vi "video server2.vi"() -> ()   [LabVIEW 2010]
doc: "Simple Data Server write a double precision array of a specified waveform type to the given TCP port. It does not provide any mechanism to halt the server or the client."
uses:
  <vilib>/userDefined/High Color/IMAQdx.ctl
  <vilib>/Utility/tcp.llb/UDP Multicast Open.vi
  <vilib>/vision/driver/NI_Vision_Acquisition_Software.lvlib
  <vilib>/vision/NI_Vision_Development_Module.lvlib
panel:
  in  "stop":bool
  in  "Multicast Address":string="234.5.6.7"
  in  "Send to Port":u16=58432
  in  "TTL":u16=1
  in  "Local Port":u16=58431
  in  "Compression (None)":i32(ring)=1 items=["None", "JPEG", "PACKED BINARY"]
  in  "Quality":i32=750 caption="Quality (750)"
  out "Image":T1(plugin-control)
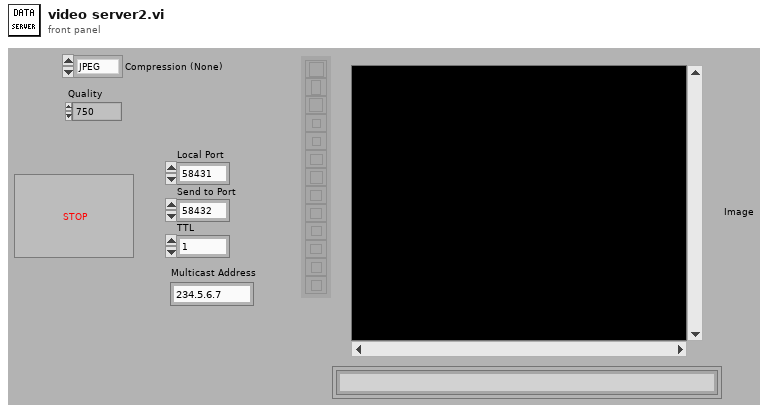
[diagram p1: front panel]
types:
  T1 = typedef "IMAQ Image.ctl" = refnum<image>
  T2 = typedef "Image Type" = u32
  T3 = typedef "IMAQdx.ctl" = refnum<k21>
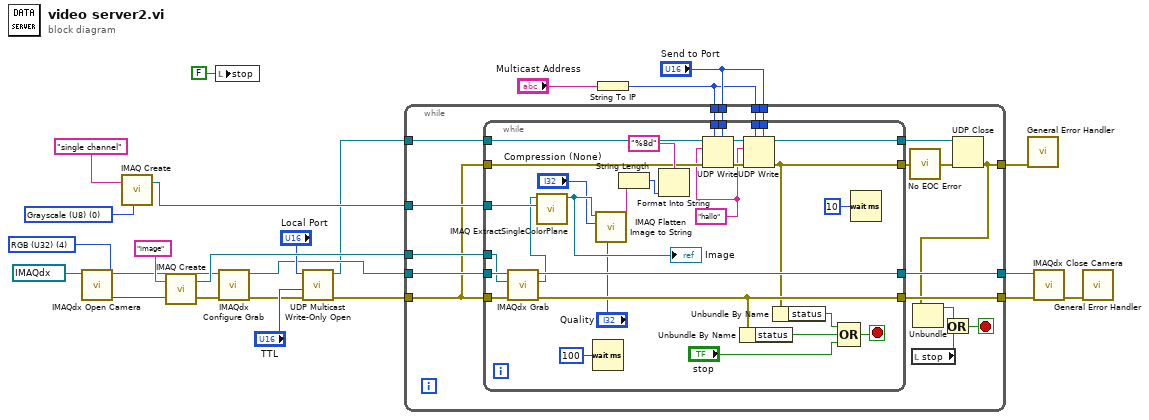
[diagram p0: block diagram]
diagram:
  w13 = T2 0 items=["Grayscale (U8)", "Grayscale (I16)", "Grayscale (SGL)", "Complex (CSG)", "RGB (U32)", "HSL (U32)", "RGB (U64)", "Grayscale (U16)"] ("Image Type")
  w21 = T2 4 items=["Grayscale (U8)", "Grayscale (I16)", "Grayscale (SGL)", "Complex (CSG)", "RGB (U32)", "HSL (U32)", "RGB (U64)", "Grayscale (U16)"] ("Image Type")
  n1 = call <vilib>:"IMAQdx Open Camera.vi"("Session In"=T3 "cam1") -> ("error out"=w19:errorcluster, "Session Out"=w20:T3)  [unwired: 9 in]
  n2 = call "IMAQ Create"("Image Name"="single channel", "Image Type"=w13) -> ("New Image"=w12:T1)  [unwired: 3 in, 1 out]
  n3 = call "IMAQ Create"("Image Name"="image", "Image Type"=w21, "error in (no error)"=w19) -> ("New Image"=w22:T1, "error out"=w18:errorcluster)  [unwired: 2 in]
  n4 = local write "stop"(FALSE ("stop")) -> ()
  n5 = call <vilib>:"IMAQdx Configure Grab.vi"("error in"=w18, "Session In"=w20) -> ("error out"=w8:errorcluster, "Session Out"=w6:T3)  [unwired: 8 in]
  n6 = call-poly <vilib>:"UDP Multicast Write-Only Open.vi"("error in (no error)"=w8, "time-to-live (1)"="TTL", "port"="Local Port") -> ("error out"=w7:errorcluster, "connection ID"=w5:refnum<k16>)  [unwired: 7 in]
  n7 = String To IP(1:"Multicast Address") -> (0:w3:u32)
  n8 = while {
    tunnel: [w33] -> w24
    tunnel: w6 -> [w41]
    tunnel: w22 -> [w40]
    tunnel: w7 -> [w35]
    tunnel: [w39] -> w17
    tunnel: [w38] -> w16
    tunnel: w12 -> [w37]
    tunnel: w5 -> [w36]
    tunnel: "Send to Port" -> [w31]
    tunnel: "Send to Port" -> [w30]
    tunnel: w3 -> [w29]
    tunnel: w3 -> [w28]
    stop <- w25 stop-if-true
    n9 = while {
      tunnel: w36 -> [w56]
      tunnel: [w51] -> w32
      tunnel: [w53] -> w42
      tunnel: w35 -> [w55]
      tunnel: w41 -> [w67]
      tunnel: w40 -> [w66]
      tunnel: w35 -> [w68]
      tunnel: [w65] -> w39
      tunnel: [w62] -> w38
      tunnel: w37 -> [w64]
      tunnel: w31 -> [w49]
      tunnel: w30 -> [w48]
      tunnel: w29 -> [w47]
      tunnel: w28 -> [w46]
      stop <- w71 stop-if-true
      w43 = "hallo" ("format string")
      n10 = call <vilib>:"IMAQdx Grab.vi"("error in"=w68, "Image In"=w66, "Session In"=w67) -> ("error out"=w62:errorcluster, "Image Out"=w63:T1, "Session Out"=w65:T3)  [unwired: 5 in, 1 out]
      n11 = call "IMAQ ExtractSingleColorPlane"("Image Dst"=w64, "Image Src"=w63) -> ("Image Dst Out"=w61:T1)  [unwired: 8 in, 1 out]
      "Image" <- w61
      n12 = Wait (ms)(milliseconds to wait=u32 100) -> ()  [unwired: 1 out]
      n13 = call "IMAQ Flatten Image to String"("Quality (750)"="Quality", "Compression (None)"="Compression (None)", "Image"=w61) -> ("Data String"=w50:string)  [unwired: 7 in, 1 out]
      n14 = String Length(string=w50) -> (length=w57:i32)
      n15 = Format Into String(format string="%8d", w57) -> ()  [unwired: 2 in, 2 out]
      n16 = UDP Write(address=w47, port or service name=w49, connection ID=w56, data in=w43, 8:w55) -> (error out=w54:errorcluster, 3:w52:refnum<k16>)  [unwired: 1 in]
      n17 = Unbundle By Name(w62) -> ("status"=w69:bool)
      n18 = UDP Write(address=w46, port or service name=w48, connection ID=w52, data in=w43, 8:w54) -> (error out=w53:errorcluster, 3:w51:refnum<k16>)  [unwired: 1 in]
      n19 = Unbundle By Name(w53) -> ("status"=w70:bool)
      n20 = Compound Arithmetic op=OR(w70, w69, "stop") -> (w71:bool)
      n21 = Wait (ms)(milliseconds to wait=u32 10) -> ()  [unwired: 1 out]
    }
    n22 = call "No EOC Error.vi"("error out 3"=w42) -> ("error out 2"=w34:errorcluster)  [unwired: 4 in]
    n23 = local read "stop"() -> (w26:bool)
    n24 = UDP Close(connection ID=w32, 8:w34) -> (error out=w33:errorcluster)  [unwired: 1 out]
    n25 = Unbundle(w33) -> ("status"=w27:bool)  [unwired: 2 out]
    n26 = Or(x=w27, y=w26) -> (x .or. y?=w25:bool)
  }
  n27 = call <vilib>:"General Error Handler.vi"("error in (no error)"=w24) -> ()  [unwired: 10 in, 5 out]
  n28 = call <vilib>:"IMAQdx Close Camera.vi"("error in"=w16, "Session In"=w17) -> ("error out"=w15:errorcluster)  [unwired: 9 in]
  n29 = call <vilib>:"General Error Handler.vi"("error in (no error)"=w15) -> ()  [unwired: 10 in, 5 out]
